vi "Paths to String with Commas.vi"(10 "Array":string[](array[string])) -> (1 "Columns":string, 2 "Table":string)   [LabVIEW 2013, in "Data.PGSQL.lvclass"]
uses:
  Data.PGSQL.lvclass
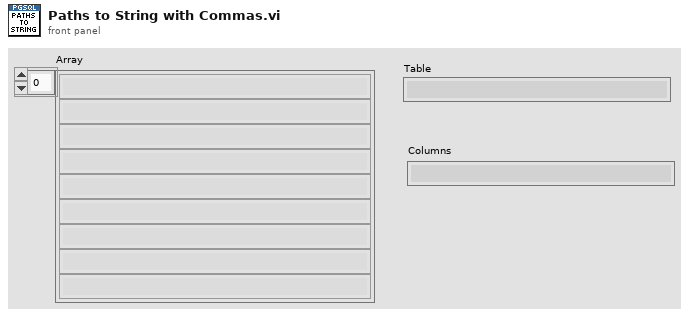
[diagram p1: front panel]
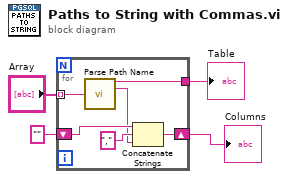
[diagram p0: block diagram]
diagram:
  n1 = for {
    shift-right: [w10] -> w4
    shift-left: "" -> [w8]
    tunnel: [w6] -> w3
    tunnel: "Array" -> [w7] mode=indexing
    n2 = call "Parse Path Name.vi"("PG Path"=w7) -> ("Table path"=w6:string, "Column path"=w5:string)  [unwired: 10 in, 3 out]
    n3 = Concatenate Strings(w8, "," ("string"), w5) -> (w10:string)
  }
  "Columns" <- w4
  "Table" <- w3
